vi "MakeSystemDefinitionPathAbsolute.vi"(8 "error in (no error)":errorcluster, 9 "relative base path":path, 11 "system definition file":path) -> (0 "error out":errorcluster, 3 "absolute system definition file":path)   [LabVIEW 2016, in "VeriStandTestCase.lvclass"]
uses:
  VeriStandTestCase.lvclass
  <userlib>/_OpenG.lib/file/file.llb/File Exists - Scalar__ogtk.vi
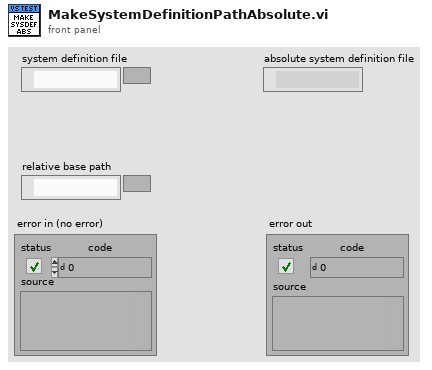
[diagram p1: front panel]
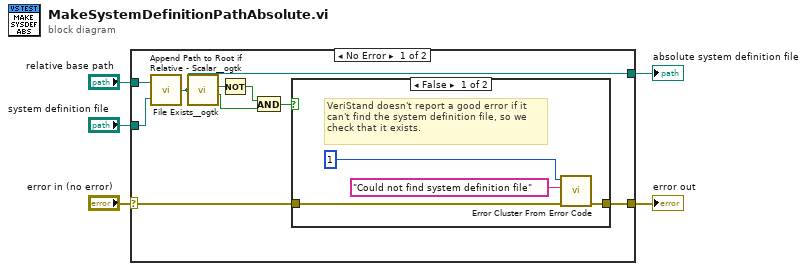
[diagram p0: block diagram]
diagram:
  n1 = case shown="No Error" "error in (no error)" {
    selector: "error in (no error)" -> [w7 w20]
    tunnel: "system definition file" -> [w14 _]
    tunnel: "relative base path" -> [w13 _]
    tunnel: [w9 _] -> w3
    tunnel: [w6 w20] -> w1
    frame No Error {
      n2 = call <userlib>:"Append Path to Root if Relative - Scalar__ogtk.vi"("Absolute or Relative Path"=w14, "Root Path"=w13) -> ("Absolute or Appended Path"=w9:path)
      n3 = call-poly <userlib>:"File Exists__ogtk.vi"("file path"=w9) -> ("is directory"=w12:bool, "exists"=w10:bool)  [unwired: 6 in]
      n4 = Not(x=w12) -> (.not. x?=w11:bool)
      n5 = And(x=w11, y=w10) -> (x .and. y?=w8:bool)
      n6 = case shown="False" w8 {
        tunnel: w7 -> [w18 w19]
        tunnel: [w17 w19] -> w6
        frame False {
          # "VeriStand doesn't report a good error if it\ncan't find the system definition file, so we\ncheck that it exists."
          n7 = call <vilib>:"Error Cluster From Error Code.vi"("error in (no error)"=w18, "error message (\"\")"="Could not find system definition file" ("error message (\"\")"), "error code (0)"=1) -> ("error out"=w17:errorcluster)  [unwired: 6 in]
        }
        frame True {
        }
      }
    }
    frame Error {
    }
  }
  "absolute system definition file" <- w3
  "error out" <- w1
